vi "Vision Research Phantom Series PhCon PhGetCameraCount.vi"(5 "Error In (no error)":errorcluster) -> (15 "pCnt":u32, 19 "Error Out":errorcluster)   [LabVIEW 2013, in "VRI.lvlib"]
doc: "PhCon.dll\n\nPhGetCameraCount\nHRESULT PhGetCameraCount(UINT *pCnt);\n\nParameters Description\npCnt (out) Return the count of cameras.\nReturn HRESULT (0=Ok)\nComments Get the count of Phantom cameras connected to this\n computer.\n If there are not cameras connected (or if you access \n a camera number above or equal to this value) the \n library switch to a simulated mode that allow you to \n test or to use the software.\n\nWritten by:\nBLOOMY CONTROLS, INC\nWINDSOR, CT 06095, USA\n860-298-9925\nwww.bloomy.com\nV1.0.0\nMay, 2004"
uses:
  VRI.lvlib
  Phantom DLLs/PhCon.dll
panel:
  # "For instructions on the use of this VI, press Ctrl+H to display the help window and move the mouse over the icon, controls, and indicators"
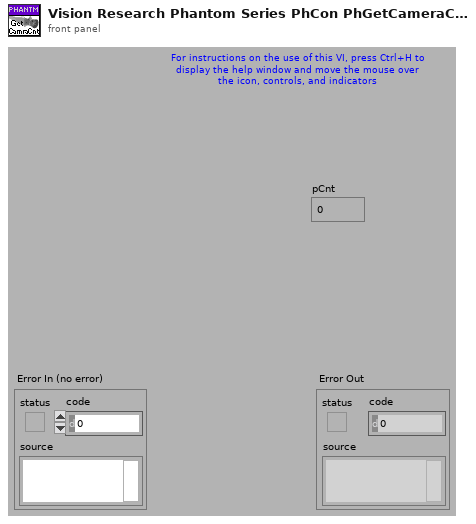
[diagram p1: front panel]
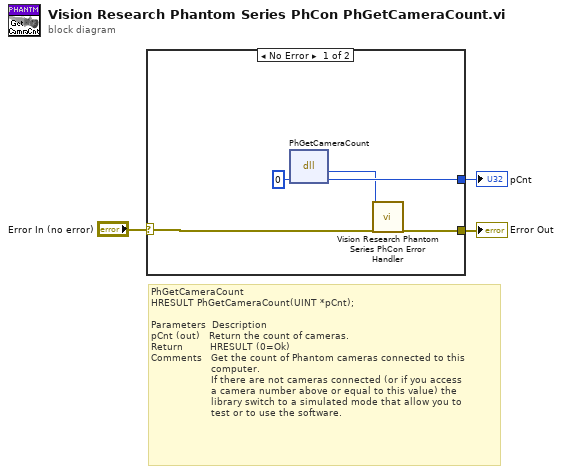
[diagram p0: block diagram]
diagram:
  # "PhGetCameraCount\nHRESULT PhGetCameraCount(UINT *pCnt);\n\nParameters  Description\npCnt (out)   Return the count of cameras.\nReturn         HRESULT (0=Ok)\nComments   Get the count of Phantom cameras connected to this\n                    computer.\n                    If there are not cameras connected (or if you access \n                    a camera number above or equal to this value) the \n                    library switch to a simulated mode that allow you to \n                    test or to use the software."
  n1 = case shown="No Error" "Error In (no error)" {
    selector: "Error In (no error)" -> [w8 w9]
    tunnel: [w7 w9] -> w2
    tunnel: [w6 _] -> w1
    frame No Error {
      n2 = dll-call lib="C:/Projects/SDK/32-bit/Vision Research Phantom Series Labview Driver/Phantom DLLs/PhCon.dll" fn="PhGetCameraCount"("pCnt"=u32 0) -> ("HRESULT"=w5:i32, "pCnt"=w6:u32)  [unwired: 3 in, 2 out]
      n3 = call "Vision Research Phantom Series PhCon Error Handler.vi"("ErrNo"=w5, "Error In (no error)"=w8) -> ("Error Out"=w7:errorcluster)  [unwired: 17 out]
    }
    frame Error {
    }
  }
  "Error Out" <- w2
  "pCnt" <- w1
